vi "07.Evd.3_Ask.4.vi"() -> ()   [LabVIEW 2025]
panel:
  out "Difference between A and B":dbl
  out "Are A and B equals?":string
  out "Larger":dbl
  out "Smaller":dbl
  in  "B":dbl
  in  "A":dbl
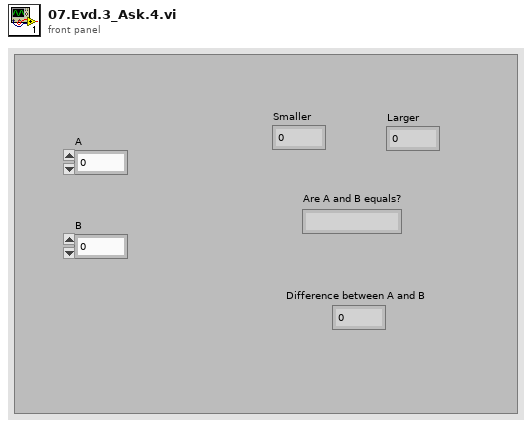
[diagram p1: front panel]
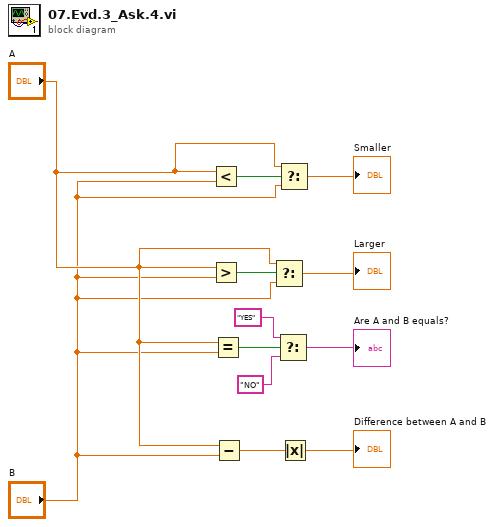
[diagram p0: block diagram]
diagram:
  n1 = Less?(x="A", y="B") -> (x < y?=w10:bool)
  n2 = Greater?(x="A", y="B") -> (0:w12:bool)
  n3 = Equal?(x="A", y="B") -> (x = y?=w5:bool)
  n4 = Subtract(x="A", y="B") -> (x-y=w8:dbl)
  n5 = Select(t="A", s=w12, f="B") -> (s? t:f=→"Larger":dbl)
  n6 = Select(t="YES", s=w5, f="NO") -> (s? t:f=→"Are A and B equals?":string)
  n7 = Select(t="A", s=w10, f="B") -> (s? t:f=→"Smaller":dbl)
  n8 = Absolute Value(x=w8) -> (abs(x)=→"Difference between A and B":dbl)
